vi "array -- bilinear regression 3D -- curvature wrapper -- V2.vi"(5 "error mode":T1=enum."errors-linear", 6 "means":T2, 8 "3D curvature tensor IN":T5={"curvature Matrix"=[[3.0, 1.0], [1.0, 4.0]], "eigenvs"=[4.618033988749895, 2.381966011250105], "Eigenvectors"=[[-0.8506508083520399+0.0i, -0.5257311121191335+0.0i], [0.5257311121191335+0.0i, -0.8506508083520399+0.0i]], "theta (rad)"=0.5535743588970453, "theta (deg)"=31.717474411461012, "Δs"=[4.618033988749895, 2.381966011250105], "δG/G"=0.5535743588970453, "Δlog(s)"=[4.618033988749895, 2.381966011250105], "inverse Matrix"=[[3.0, 1.0], [1.0, 4.0]], "noise T"=0.5535743588970453} {"noise T" format="%#_3f"; "inverse Matrix" format="%#_3p"; "Δlog(s)" scale=0.001..10.0; "δG/G" format="%#_3f"; "Δs" format="%#_2p"; "theta (deg)" format="%#_3p"; "curvature Matrix" format="%#_3p"; "eigenvs" format="%#_2f"; "Eigenvectors" format="%#_3p"; "theta (rad)" format="%#_3p"}, 9 "fit map IN":map{T4, dbl}(c390), 11 "xyzw  IN":T3={"x"=[-2.0, -1.0, 0.0, 1.0, 2.0], "y"=[-2.0, -1.0, 0.0, 1.0, 2.0], "w"=[-2.0, -1.0, 0.0, 1.0, 2.0], "z"=[12.0, 3.0, 0.0, 3.0, 12.0]}) -> (0 "3D curvature tensor OUT":T5={"curvature Matrix"=[[0.9999999999999996, 0.9999999999999998], [0.9999999999999998, 1.0]], "eigenvs"=[1.7838428397948585, 0.21615716020514097], "Eigenvectors"=[[-0.8506508083520399+0.0i, -0.5257311121191335+0.0i], [0.5257311121191335+0.0i, -0.8506508083520399+0.0i]], "theta (rad)"=0.7853981633974482, "theta (deg)"=44.99999999999999, "Δs"=[nan, nan], "δG/G"=0.5535743588970453, "Δlog(s)"=[4.618033988749895, 2.381966011250105], "inverse Matrix"=[], "noise T"=0.5535743588970453} {"noise T" format="%#_3f"; "inverse Matrix" format="%#_3p"; "Δlog(s)" scale=0.001..10.0; "δG/G" format="%#_3f"; "Δs" format="%#_2p"; "theta (deg)" format="%#_3p"; "curvature Matrix" format="%#_3p"; "eigenvs" format="%#_2f"; "Eigenvectors" format="%#_3p"; "theta (rad)" format="%#_3p"}, 1 "fit map out":map{T4, dbl}(c390), 3 "xyzw  OUT":T3={"x"=[-2.0, -1.0, 0.0, 1.0, 2.0], "y"=[-2.0, -1.0, 0.0, 1.0, 2.0], "w"=[-2.0, -1.0, 0.0, 1.0, 2.0], "z"=[12.0, 3.0, 0.0, 3.0, 12.0]})   [LabVIEW 2021]
uses:
  array -- bilinear regression 2D.ctl
  <vilib>/Analysis/Matrix/Datatypes/RealMatrix.ctl
  3D curvature tensor.ctl
  <vilib>/Analysis/Matrix/Datatypes/ComplexMatrix.ctl
  4-vec-array.ctl
  3-vec.ctl
  nanocal generate curvature ellipse -- action.ctl
  array -- fit control .ctl
  2D curvature tensor actions.ctl
  <vilib>/Analysis/7linalg.llb/Solve Linear Equations.vi
  <vilib>/Analysis/7linalg.llb/Solve Linear Equations (single right hand).vi
  array -- linear regression 3D -- V2.vi
  <vilib>/Analysis/baseanly.llb/A x B.vi
  <vilib>/Analysis/baseanly.llb/Real A x B.vi
  <vilib>/Analysis/baseanly.llb/Solve Linear Equations By Cholesky.vi
  <vilib>/Analysis/baseanly.llb/Real Matrix to Compact Array.vi
  <vilib>/Analysis/baseanly.llb/Real Compact Tri-Matrix Linear Eqs.vi
  <vilib>/Analysis/Matrix/Numeric/Conversions/Array To Matrix - RA2.vi
  <vilib>/Analysis/7linalg.llb/Solve Linear Eqs (General).vi
  <vilib>/Analysis/7linalg.llb/Solve Linear Eqs (Gen, single right hand).vi
  <vilib>/Analysis/Matrix/Numeric/Conversions/Matrix To Array.vi
  <vilib>/Analysis/Matrix/Numeric/Conversions/Matrix To Array - RM.vi
  <vilib>/Analysis/7linalg.llb/Eigenvalues and Vectors.vi
  <vilib>/Analysis/7linalg.llb/Real Eigenvalues and Vectors.vi
  <vilib>/Analysis/baseanly.llb/Inverse Matrix.vi
  <vilib>/Analysis/baseanly.llb/Real Inverse Matrix.vi
  <vilib>/Analysis/Matrix/NI_Matrix.lvlib
panel:
  out "curvature Matrix":T6=[[0.9999999999999996, 0.9999999999999998], [0.9999999999999998, 1.0]]
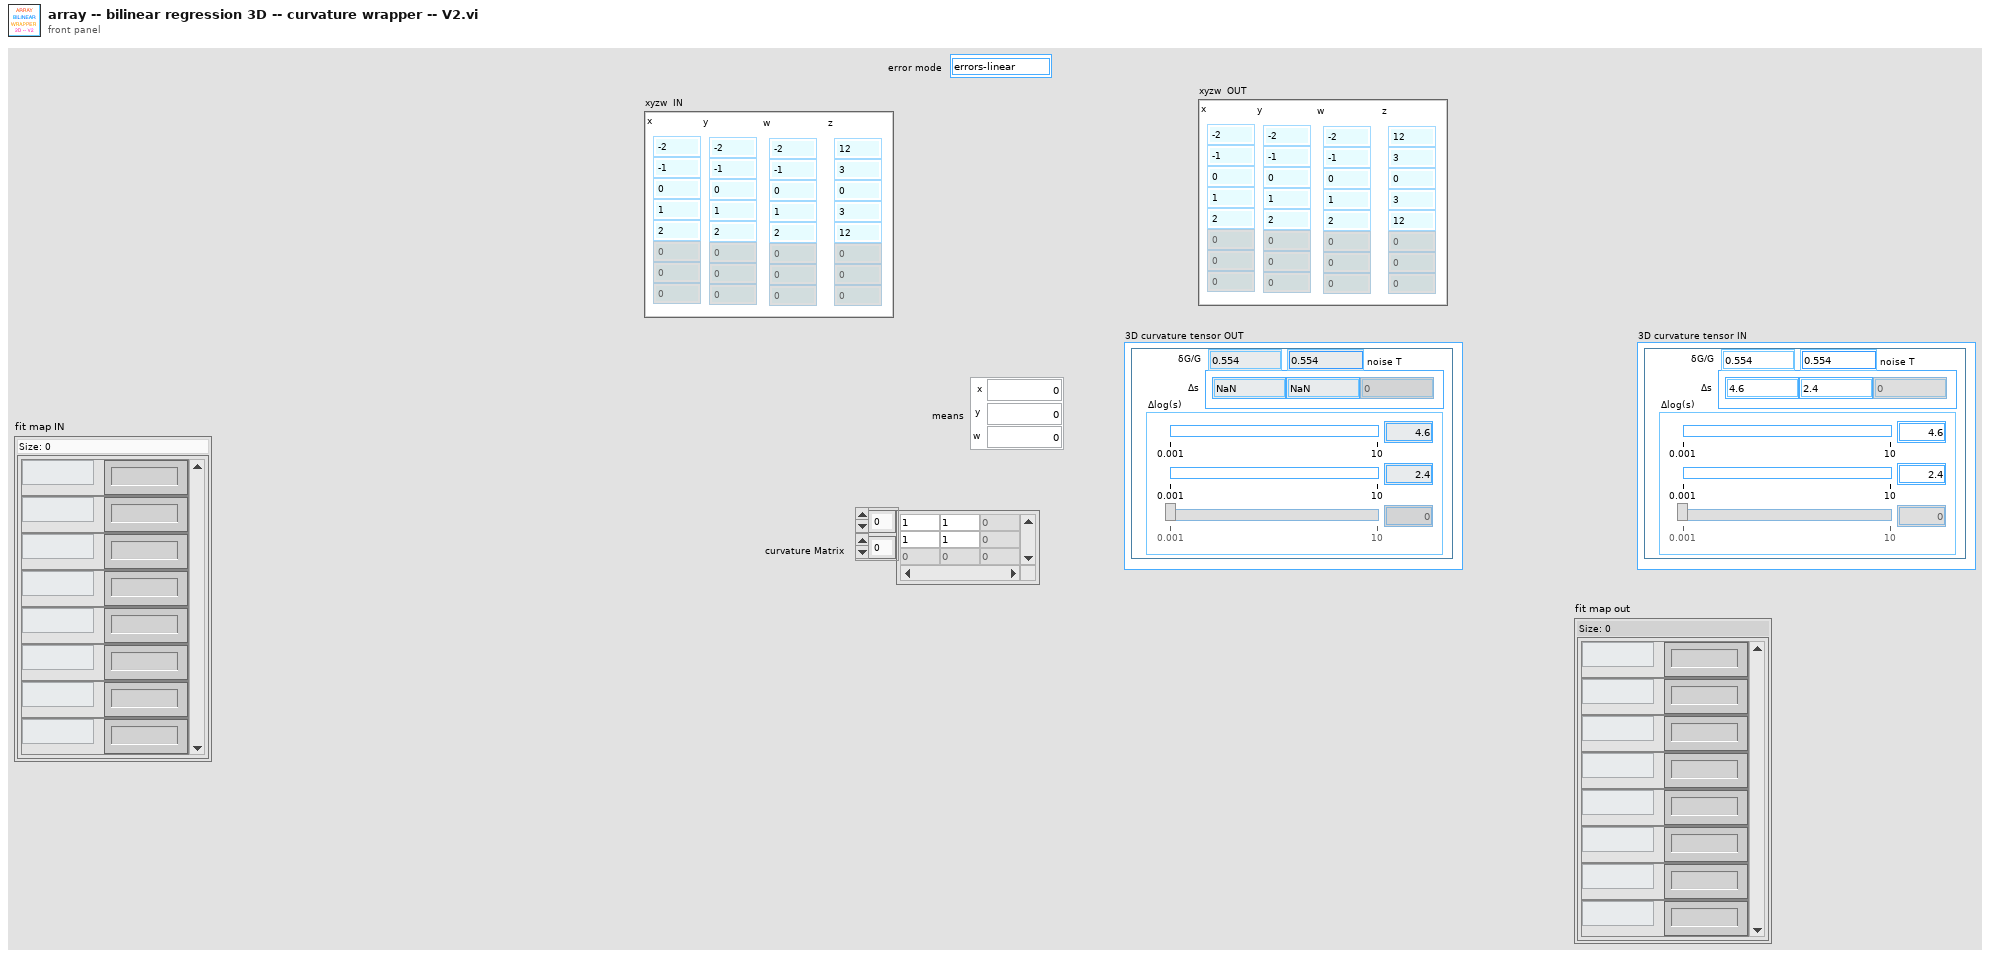
[diagram p1: front panel]
types:
  T1 = typedef "nanocal generate curvature ellipse -- action.ctl" = enum16{"errors-log", "errors-linear"}
  T2 = typedef "3-vec.ctl" = cluster{"x":dbl, "y":dbl, "w":dbl}
  T3 = typedef "4-vec-array.ctl" = cluster{"x":dbl[], "y":dbl[], "w":dbl[], "z":dbl[]}
  T4 = typedef "array -- bilinear regression 2D.ctl" = enum16{"1", "x", "y", "xx", "xy", "yy", "xxy", "xyy", "yyy", "xxx", "xxyy", "xyyy", "xxxy", "yyyy", "xxxx", "xxz", "xyz", "yyz", "xz", "yz", "z", "wwz", "ywz", "xwz", "xxxw", "xxyw", "xyyw", "yyyw", "xxww", "xyww", "yyww", "xwww", "ywww", "wwww", "ww", "xw", "yw", "w", "wz", "xxw", "yyw", "xyw", "xww", "yww", "www"}
  T5 = typedef "3D curvature tensor.ctl" = cluster{"curvature Matrix":T6, "eigenvs":dbl[], "Eigenvectors":T7, "theta (rad)":dbl, "theta (deg)":dbl, "Δs":dbl[], "δG/G":dbl, "Δlog(s)":dbl[], "inverse Matrix":T6, "noise T":dbl}
  T6 = typedef "NI_Matrix.lvlib/RealMatrix.ctl" = dbl[][]
  T7 = typedef "NI_Matrix.lvlib/ComplexMatrix.ctl" = cdb[][]
  T8 = typedef "array -- fit control .ctl" = enum16{"fit", "calc", "check", "init"}
  T9 = typedef "2D curvature tensor actions.ctl" = enum16{"eigensystem", "sigma", "set matrix", "inverse"}
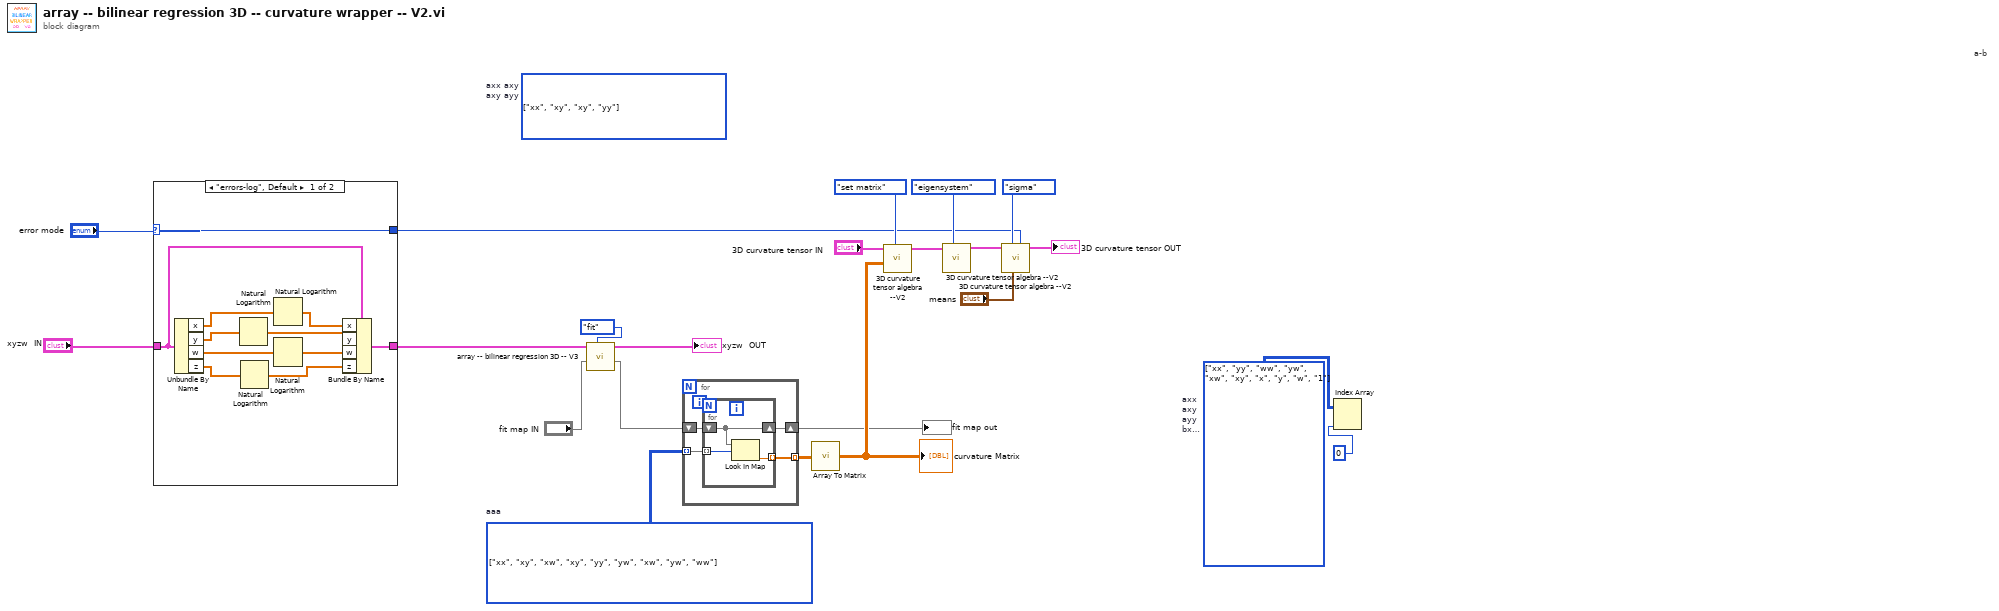
[diagram p0: block diagram]
diagram:
  w10 = T4[][] [[enum."xx", enum."xy", enum."xw"], [enum."xy", enum."yy", enum."yw"], [enum."xw", enum."yw", enum."ww"]] items=["1", "x", "y", "xx", "xy", "yy", "xxy", "xyy", "yyy", "xxx", "xxyy", "xyyy", "xxxy", "yyyy", "xxxx", "xxz", "xyz", "yyz", "xz", "yz", "z", "wwz", "ywz", "xwz", "xxxw", "xxyw", "xyyw", "yyyw", "xxww", "xyww", "yyww", "xwww", "ywww", "wwww", "ww", "xw", "yw", "w", "wz", "xxw", "yyw", "xyw", "xww", "yww", "www"]  # aaa
  w12 = T4[][] [[enum."xx"], [enum."yy"], [enum."ww"], [enum."yw"], [enum."xw"], [enum."xy"], [enum."x"], [enum."y"], [enum."w"], [enum."1"]] items=["1", "x", "y", "xx", "xy", "yy", "xxy", "xyy", "yyy", "xxx", "xxyy", "xyyy", "xxxy", "yyyy", "xxxx", "xxz", "xyz", "yyz", "xz", "yz", "z", "wwz", "ywz", "xwz", "xxxw", "xxyw", "xyyw", "yyyw", "xxww", "xyww", "yyww", "xwww", "ywww", "wwww", "ww", "xw", "yw", "w", "wz", "xxw", "yyw", "xyw", "xww", "yww", "www"]  # axx axy ayy bx by c
  (unwired) T4[][] [[enum."xx", enum."xy"], [enum."xy", enum."yy"]] items=["1", "x", "y", "xx", "xy", "yy", "xxy", "xyy", "yyy", "xxx", "xxyy", "xyyy", "xxxy", "yyyy", "xxxx", "xxz", "xyz", "yyz", "xz", "yz", "z", "wwz", "ywz", "xwz", "xxxw", "xxyw", "xyyw", "yyyw", "xxww", "xyww", "yyww", "xwww", "ywww", "wwww", "ww", "xw", "yw", "w", "wz", "xxw", "yyw", "xyw", "xww", "yww", "www"]  # axx axy axy ayy
  # "a-b"
  n1 = case shown="\"errors-log\", Default" "error mode" {
    selector: "error mode" -> [w33 w34]
    tunnel: "xyzw  IN" -> [w32 w35]
    tunnel: [w23 w35] -> w3
    tunnel: [w33 w34] -> w1
    frame "errors-log", Default {
      n2 = Unbundle By Name(w32) -> ("x"=w31:dbl[], "y"=w29:dbl[], "w"=w24:dbl[], "z"=w25:dbl[])
      n3 = Natural Logarithm(1:w29) -> (0:w28:dbl[])
      n4 = Natural Logarithm(1:w25) -> (0:w26:dbl[])
      n5 = Natural Logarithm(1:w31) -> (0:w30:dbl[])
      n6 = Natural Logarithm(1:w24) -> (0:w27:dbl[])
      n7 = Bundle By Name(cluster=w32, "x"=w30, "y"=w28, "w"=w27, "z"=w26) -> (w23:T3)
    }
    frame "errors-linear" {
    }
  }
  n8 = call "array -- bilinear regression 3D -- V3.vi"("action"=array_--_fit_control_."fit", "fit map IN"="fit map IN", "xyzw IN"=w3) -> ("fit map out"=w13:map{T4, dbl}, "xyzw OUT"=→"xyzw  OUT":T3)  [unwired: 7 in]
  n9 = for {
    tunnel: w10 -> [w39] mode=indexing
    shift-right: [w37] -> w9
    shift-left: w13 -> [w38]
    tunnel: [w36] -> w22 mode=indexing
    n10 = for {
      tunnel: w39 -> [w41] mode=indexing
      shift-right: [w42] -> w37
      shift-left: w38 -> [w42]
      tunnel: [w40] -> w36 mode=indexing
      n11 = Look In Map(map=w42, key=w41) -> (value=w40:dbl)  [unwired: 1 in, 1 out]
    }
  }
  "fit map out" <- w9
  n12 = call-poly <vilib>:"Array To Matrix.vi"("Real 2D Array"=w22) -> ("Real Matrix"=w18:T6)
  "curvature Matrix" <- w18
  n13 = call "3D curvature tensor algebra --V2.vi"("2D tensor action"=2D_curvature_tensor_actions."set matrix" ("2D tensor"), "3D curvature Matrix IN"=w18, "3D curvature tensor IN"="3D curvature tensor IN") -> ("3D curvature tensor OUT"=w20:T5)  [unwired: 7 in, 1 out]
  n14 = call "3D curvature tensor algebra --V2.vi"("2D tensor action"=2D_curvature_tensor_actions."eigensystem" ("2D tensor"), "3D curvature tensor IN"=w20) -> ("3D curvature tensor OUT"=w17:T5)  [unwired: 8 in, 1 out]
  n15 = call "3D curvature tensor algebra --V2.vi"("error mode"=w1, "means"="means", "2D tensor action"=2D_curvature_tensor_actions."sigma" ("2D tensor"), "3D curvature tensor IN"=w17) -> ("3D curvature tensor OUT"=→"3D curvature tensor OUT":T5)  [unwired: 6 in, 1 out]
  n16 = Index Array(array=w12, index (col)=0 ("disabled index (col)")) -> ()  [unwired: 1 in, 1 out]
